vi "Update Tree Symbol.vi"(4 "method type":enum16{"setUp", "testMethod", "tearDown"}(ring), 5 "test error":errorcluster, 6 "resultStatus":T1(ring), 7 "SuitesRunning":string[](array[string]), 8 "error in":errorcluster, 9 "IsTestCase":bool, 10 "test GUID":string, 11 "Test Hierarchy Tree":refnum<vi>) -> ()   [LabVIEW 2011, in "GraphicalTestRunner.lvlib"]
uses:
  GraphicalTestRunner.lvlib
  JKI Reuse/Filter Error Codes (Scalar)__jki_lib_error_handling -- VI Tester.vi
  <userlib>/_OpenG.lib/string/string.llb/Convert EOLs (String)__ogtk.vi
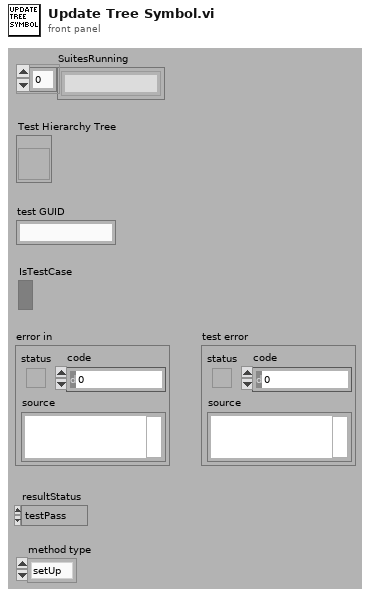
[diagram p1: front panel]
types:
  T1 = enum16{"testPass", "testFailure", "testError", "testSkipped"}
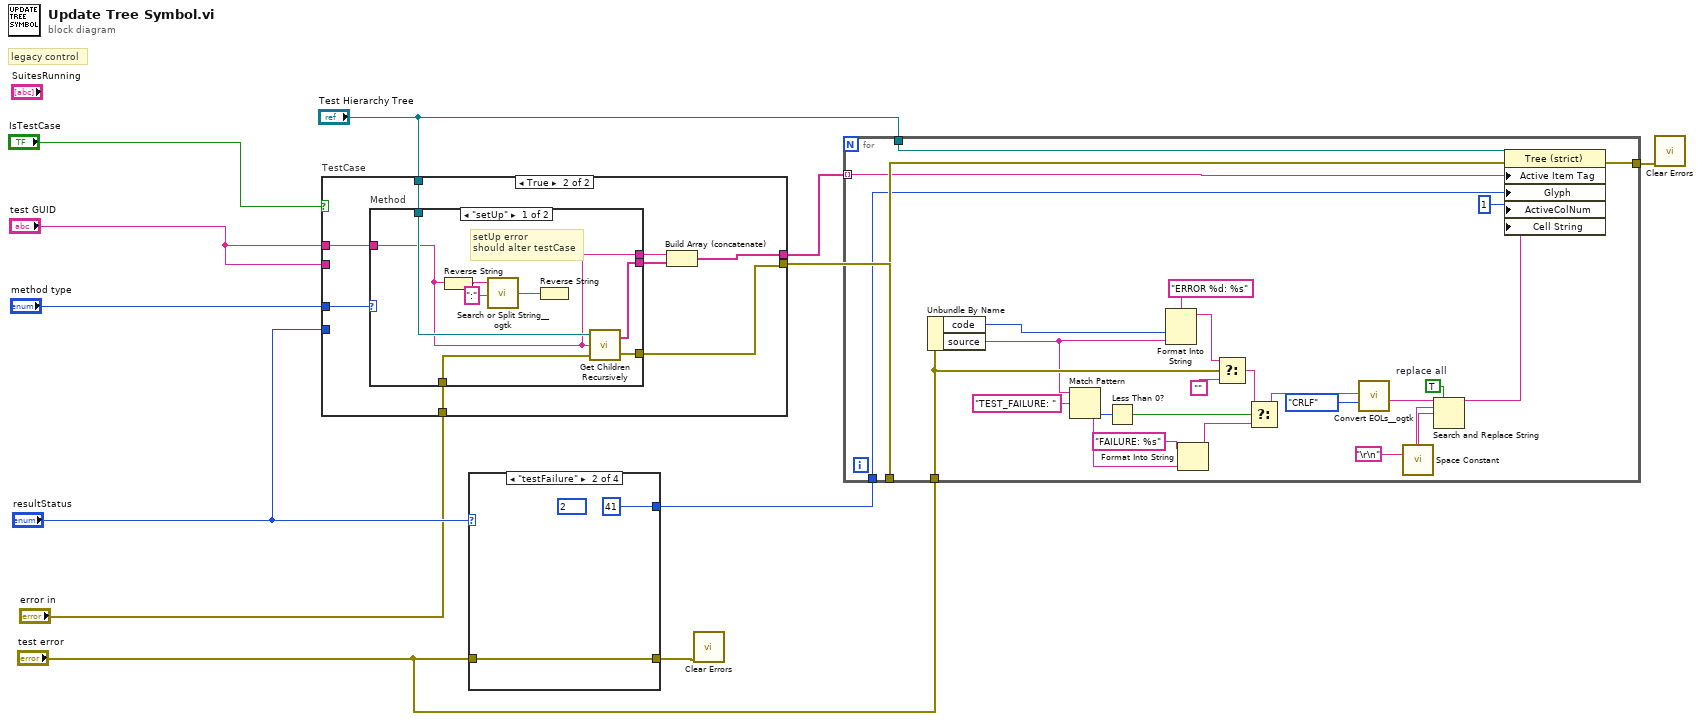
[diagram p0: block diagram]
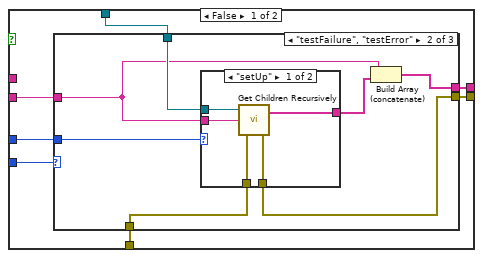
[diagram p2: hidden frame]
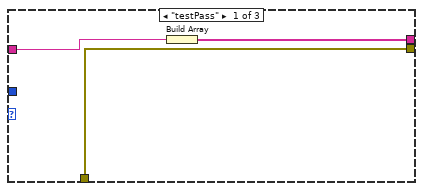
[diagram p3: hidden frame]
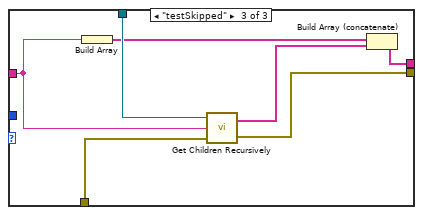
[diagram p5: hidden frame]
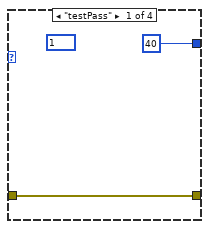
[diagram p7: hidden frame]
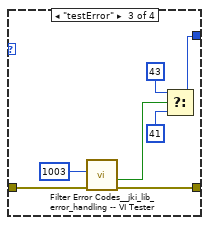
[diagram p8: hidden frame]
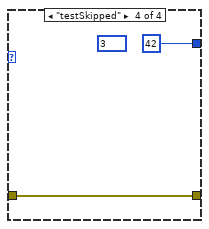
[diagram p9: hidden frame]
diagram:
  # "legacy control"
  n1 = case "TestCase" shown="True" "IsTestCase" {
    tunnel: "test GUID" -> [w17 _]
    tunnel: "test GUID" -> [_ w49]
    tunnel: [w14 w47] -> w10
    tunnel: "method type" -> [w13 w50]
    tunnel: "resultStatus" -> [w19 _]
    tunnel: "Test Hierarchy Tree" -> [w18 w46]
    tunnel: "error in" -> [w16 w44]
    tunnel: [w15 w43] -> w3
    frame False {
      n2 = case shown="\"testFailure\", \"testError\"" w19 {
        tunnel: w18 -> [_ w28 w42]
        tunnel: w17 -> [w21 w25 w36]
        tunnel: w16 -> [w22 w27 w41]
        tunnel: [w22 w26 w40] -> w15
        tunnel: [w20 w24 w38] -> w14
        tunnel: w13 -> [_ w29 _]
        frame "testPass" {
          n3 = Build Array(w21) -> (w20:string[])
        }
        frame "testFailure", "testError" {
          n4 = case shown="\"setUp\"" w29 {
            tunnel: w25 -> [w31 _]
            tunnel: [w30 _] -> w23
            tunnel: w28 -> [w34 _]
            tunnel: w27 -> [w33 w35]
            tunnel: [w32 w35] -> w26
            frame "setUp" {
              n5 = call "Get Children Recursively.vi"("error in"=w33, "Parent"=w31, "Tree"=w34) -> ("error out"=w32:errorcluster, "Recursive Children"=w30:string[])
            }
            frame "testMethod", Default {
            }
          }
          n6 = Build Array (concatenate)(w25, w23) -> (w24:string[])
        }
        frame "testSkipped" {
          n7 = Build Array(w36) -> (w39:string[])
          n8 = call "Get Children Recursively.vi"("error in"=w41, "Parent"=w36, "Tree"=w42) -> ("error out"=w40:errorcluster, "Recursive Children"=w37:string[])
          n9 = Build Array (concatenate)(w39, w37) -> (w38:string[])
        }
      }
    }
    frame True {
      n10 = case "Method" shown="\"setUp\"" w50 {
        tunnel: w49 -> [w51 w60]
        tunnel: [w51 w60] -> w48
        tunnel: w46 -> [w55 _]
        tunnel: [w54 _] -> w45
        tunnel: w44 -> [w53 w59]
        tunnel: [w52 w59] -> w43
        frame "setUp" {
          # "setUp error\nshould alter testCase"
          n11 = Reverse String(1:w51) -> (0:w58:string)
          n12 = call <userlib>:"Search or Split String__ogtk.vi"("search string/char (-)"=":", "string"=w58) -> ("substring after match"=w56:string)  [unwired: 1 in, 2 out]
          n13 = Reverse String(1:w56) -> ()  [unwired: 1 out]
          n14 = call "Get Children Recursively.vi"("error in"=w53, "Parent"=w51, "Tree"=w55) -> ("error out"=w52:errorcluster, "Recursive Children"=w54:string[])
        }
        frame "testMethod", Default {
        }
      }
      n15 = Build Array (concatenate)(w48, w45) -> (w47:string[])
    }
  }
  n16 = case shown="\"testFailure\"" "resultStatus" {
    tunnel: [40 41 w67 42] -> w9
    tunnel: "test error" -> [w61 w63 w70 w72]
    tunnel: [w61 w63 w65 w72] -> w2
    frame "testPass" {
      (unwired) 1
    }
    frame "testFailure" {
      (unwired) 2
    }
    frame "testError" {
      n17 = call-poly "Filter Error Codes__jki_lib_error_handling -- VI Tester.vi"("error in"=w70, "error code to filter"=1003) -> ("error out"=w65:errorcluster, "error filtered?"=w69:bool)  [unwired: 7 in, 1 out]
      n18 = Select(t=43, s=w69, f=41) -> (s? t:f=w67:i32)
    }
    frame "testSkipped" {
      (unwired) 3
    }
  }
  n19 = call <vilib>:"Clear Errors.vi"("error in (no error)"=w2) -> ()  [unwired: 6 in, 1 out]
  n20 = for {
    tunnel: w3 -> [w99]
    tunnel: "Test Hierarchy Tree" -> [w98]
    tunnel: [w97] -> w12
    tunnel: w10 -> [w96] mode=indexing
    tunnel: w9 -> [w95]
    tunnel: "test error" -> [w78]
    w91 = TRUE  # replace all
    n21 = Unbundle By Name(w78) -> ("code"=w79:i32, "source"=w74:string)
    n22 = Match Pattern(string=w74, regular expression="TEST_FAILURE: ") -> (after substring=w81:string, offset past match=w86:i32)  [unwired: 1 in, 2 out]
    n23 = Less Than 0?(x=w86) -> (x < 0?=w85:bool)
    n24 = Format Into String(format string="ERROR %d: %s", w79, w74) -> (resulting string=w76:string)  [unwired: 2 in, 1 out]
    n25 = Format Into String(format string="FAILURE: %s", w81) -> (resulting string=w83:string)  [unwired: 2 in, 1 out]
    n26 = Select(t=w76, s=w78, f="") -> (s? t:f=w75:string)
    n27 = Select(t=w75, s=w85, f=w83) -> (s? t:f=w80:string)
    n28 = call-poly <userlib>:"Convert EOLs__ogtk.vi"("Convert to:"=enum16{"CR", "LF", "CRLF"}."CRLF", "String in"=w80) -> ("String out"=w92:string)  [unwired: 9 in]
    n29 = call <vilib>:"Space Constant.vi"() -> ("String"=w89:string)
    n30 = Search and Replace String(replace all?=w91, input string=w92, search string="\r\n", replace string=w89) -> (result string=w88:string)  [unwired: 4 in, 3 out]
    n31 = property class="Tree (strict)"(reference=w98, error in=w99, "Active Item Tag"=w96, "Glyph"=w95, "ActiveColNum"=1 ("Active Cell:Active Column Number"), "Cell String"=w88) -> (error out=w97:errorcluster)  [unwired: 1 out]
  }
  n32 = call <vilib>:"Clear Errors.vi"("error in (no error)"=w12) -> ()  [unwired: 6 in, 1 out]
